vi "To RGBA.vi"(10 "Depth":i32, 11 "Image Data":u8[](array[numeric])) -> (3 "RGBA":u8[](array[numeric]))   [LabVIEW 2020, in "G-Image.lvlib"]
doc: "Convert the image memory layout from RGB or ARGB to RGBA. Applies to 24-bit and 32-bit images only."
uses:
  G-Image.lvlib
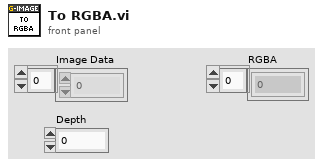
[diagram p1: front panel]
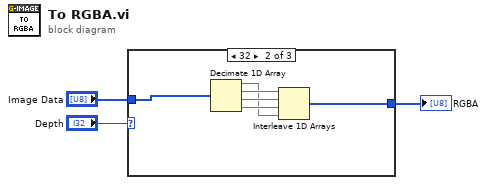
[diagram p0: block diagram]
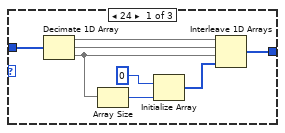
[diagram p2: hidden frame]
diagram:
  n1 = case shown="32" "Depth" {
    tunnel: "Image Data" -> [w11 w17 w18]
    tunnel: [w10 w16 w18] -> w1
    frame 24 {
      n2 = Decimate 1D Array(w11) -> (w9:u8[], w8:u8[], w6:u8[])
      n3 = Array Size(array=w6) -> (size(s)=w7:i32)
      n4 = Initialize Array(u8 0, w7) -> (w4:u8[])
      n5 = Interleave 1D Arrays(w9, w8, w6, w4) -> (w10:u8[])
    }
    frame 32 {
      n6 = Decimate 1D Array(w17) -> (w12:u8[], w15:u8[], w14:u8[], w13:u8[])
      n7 = Interleave 1D Arrays(w15, w14, w13, w12) -> (w16:u8[])
    }
    frame Default {
      # "1, 4, 8, 32"
    }
  }
  "RGBA" <- w1
